vi "Initialize.vi"(8 "error in (no error)":errorcluster, 11 "DVR_Waveforms (N Ch).lvclass":refnum<class "Waveforms (N Ch).lvclass">) -> (0 "error out":errorcluster, 3 "DVR_Waveforms (N Ch).lvclass":refnum<class "Waveforms (N Ch).lvclass">)   [LabVIEW 2017, in "Waveforms (N Ch).lvclass"]
uses:
  <vilib>/addons/_NISVFA/_Shared subVIs/Data Objects/Waveforms (DBL)/Waveforms (N Ch).lvclass
  C:/Program Files (x86)/National Instruments/LabVIEW 2017/vi.lib/addons/_NISVFA/_Shared subVIs/Data Objects/Data/Data.lvclass
  <vilib>/addons/_NISVFA/_Shared subVIs/Data Objects/Data/Data.lvclass/Data.ctl
  <vilib>/addons/_NISVFA/_Shared subVIs/Data Objects/Data/Read Data Attributes.vi
  <vilib>/addons/_NISVFA/_Shared subVIs/Data Objects/Data/Data.lvclass
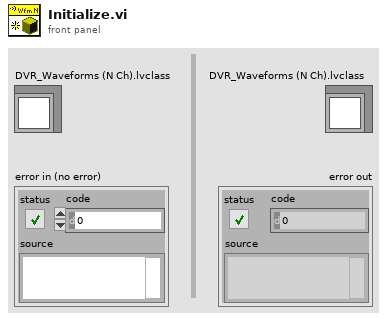
[diagram p1: front panel]
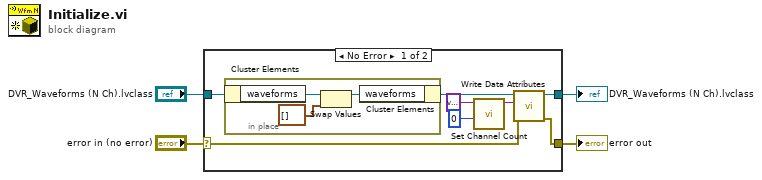
[diagram p0: block diagram]
diagram:
  n1 = case shown="No Error" "error in (no error)" {
    selector: "error in (no error)" -> [w11 w16]
    tunnel: "DVR_Waveforms (N Ch).lvclass" -> [w9 w15]
    tunnel: [w8 w15] -> w4
    tunnel: [w10 w16] -> w2
    frame No Error {
      n2 = in-place {
        n3 = in-place-cluster #1(w9) -> ("waveforms"=w13:waveform(dbl)[])
        n4 = Swap Values(12:w13, 14:waveform(dbl)[] [] ("waveforms")) -> (1:w12:waveform(dbl)[])  [unwired: 1 in, 1 out]
        n5 = in-place-cluster #1("waveforms"=w12) -> ()  [unwired: 1 out]
      }
      n6 = call <vilib>:"Set Channel Count.vi"("number of channels"=0, "variant in"=variant ("data attributes")) -> ("variant out"=w6:variant)  [unwired: 9 in]
      n7 = call <vilib>:"Write Data Attributes.vi"("error in (no error)"=w11, "data attributes"=w6, "Data in"=w9) -> ("error out"=w10:errorcluster, "Data out"=w8:refnum<class "Waveforms (N Ch).lvclass">)  [unwired: 7 in]
    }
    frame Error {
    }
  }
  "DVR_Waveforms (N Ch).lvclass" <- w4
  "error out" <- w2
